vi "Initial Values-format and values-ROI window.vi"() -> (13 "Values.Boolean":bool[](array[boolean]), 14 "Keys setup.DBL":T2=[{"key"="Control FPGA.Clock Freq (MHz)", "Save?"=TRUE, "Default"=240.0}, {"key"="DAQ FPGA.Clock Freq (MHz)", "Save?"=TRUE, "Default"=240.0}], 15 "Values.DBL":dbl[](array[numeric]), 16 "Keys setup.String":T3=[{"key"="Control FPGA.MAC address", "Save?"=TRUE, "Default"="AABBCCDDEEFF"}, {"key"="DAQ FPGA.Target", "Save?"=TRUE, "Default"="RIO0"}, {"key"="XY Stage.COM port", "Save?"=TRUE, "Default"="COM7"}, {"key"="DAQmx Chan.Pockels Control", "Save?"=TRUE, "Default"=""}, {"key"="DAQmx Chan.Hard Shutter", "Save?"=TRUE, "Default"=""}, {"key"="DAQmx Chan.PMT 1", "Save?"=TRUE, "Default"=""}, {"key"="DAQmx Chan.PMT 2", "Save?"=TRUE, "Default"=""}, {"key"="DAQmx Chan.Encoder Trigger", "Save?"=TRUE, "Default"=""}, {"key"="DAQmx Chan.Optional Trigger 1", "Save?"=TRUE, "Default"=""}, {"key"="DAQmx Chan.Optional Trigger 2", "Save?"=TRUE, "Default"=""}, {"key"="DAQmx Chan.Optional Trigger 3", "Save?"=TRUE, "Default"=""}], 17 "Values.Strings":string[](array[string]), 18 "Keys setup.Boolean":T1, 19 "error out":errorcluster)   [LabVIEW 2020]
uses:
  Typedefs/Ini file interface (String).ctl
  Typedefs/Ini file interface (DBL).ctl
  Typedefs/Ini file interface (Boolean).ctl
  User Interface/ROI Entry screen/Globals/gl_ROI Entry UI globals.vi
panel:
  # "NOTES:\n1. \"Control FPGA.Ethernet port\" is detected automatically. It is not saved/loaded from file.\n2. \"Control FPGA.Ethernet Opened\" is detected automatically. It is not saved/loaded from file."
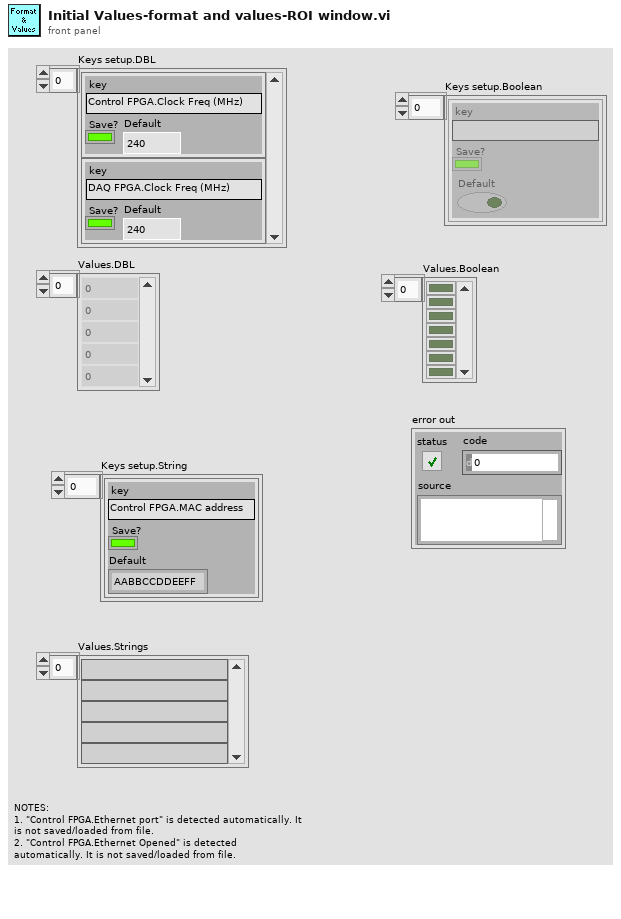
[diagram p1: front panel]
types:
  T1 = typedef "Ini file interface (Boolean).ctl" = cluster{"key":string, "Save?":bool, "Default":bool}[]
  T2 = typedef "Ini file interface (DBL).ctl" = cluster{"key":string, "Save?":bool, "Default":dbl}[]
  T3 = typedef "Ini file interface (String).ctl" = cluster{"key":string, "Save?":bool, "Default":string}[]
  T4 = typedef "ROI entry screen ctrl refs cluster.ctl" = cluster{"Done button":refnum<vi>, "Imaging button":refnum<vi>, "Acquisition button":refnum<vi>, "Scan dwell time per pixel (us)":refnum<vi>, "# of planes":refnum<vi>, "Zoom Ctrl":refnum<vi>, "Equal size":refnum<vi>, "Channel":refnum<vi>, "Image Display":refnum<vi>, "Z-Plane Selector":refnum<vi>, "Number of lines left":refnum<vi>, "Z-stack folder path":refnum<vi>, "POI Density":refnum<vi>, "Arb Plane Entry":refnum<vi>, "Whole Plane":refnum<vi>, "Line Mode":refnum<vi>, "Clear Last":refnum<vi>, "Clear All":refnum<vi>, "Delete Lines":refnum<vi>, "Trial Length (sec)":refnum<vi>, "Palette Type":refnum<vi>, "Intensity slider":refnum<vi>, "# POI":refnum<vi>, "Max Z Proj":refnum<vi>, "Zplane ind":refnum<vi>, "Wavelength (nm)":refnum<vi>, "Number of Trials":refnum<vi>, "Funct stim.trig.enable":refnum<vi>, "Funct stim.trig.delay (s)":refnum<vi>, "Line Mode":refnum<vi>, "Step size (µm)":refnum<vi>, "ROI move mode":refnum<vi>, "Cool-down time (s)":refnum<vi>, "Enable cool-down time":refnum<vi>, "Motor Z ind. (um)":refnum<vi>, "AOL Z ind. (um)":refnum<vi>, "Load Reference Image":refnum<vi>, "Rel.  Res.":refnum<vi>, "ROI LIST":refnum<vi>, "Show All":refnum<vi>, "ROI Type":refnum<vi>, "Start Plane":refnum<vi>, "Stop Plane":refnum<vi>, "Offset ROI":refnum<vi>, "Tab Control":refnum<vi>, "Laser Power(%)":refnum<vi>, "Cycle rate":refnum<vi>, "FOV (Ind.)":refnum<vi>, "Frame Size (Ind.)":refnum<vi>, "Resolution (Ind.)":refnum<vi>, "Pixel Density (Ind)":refnum<vi>, "Laser Power (Ind.)":refnum<vi>, "Dwell Time (Ind.)":refnum<vi>, "Adj MC":refnum<vi>}
  T5 = enum16{"Grayscale", "Binary", "Gradient", "Rainbow", "Temperature", "User Defined"}
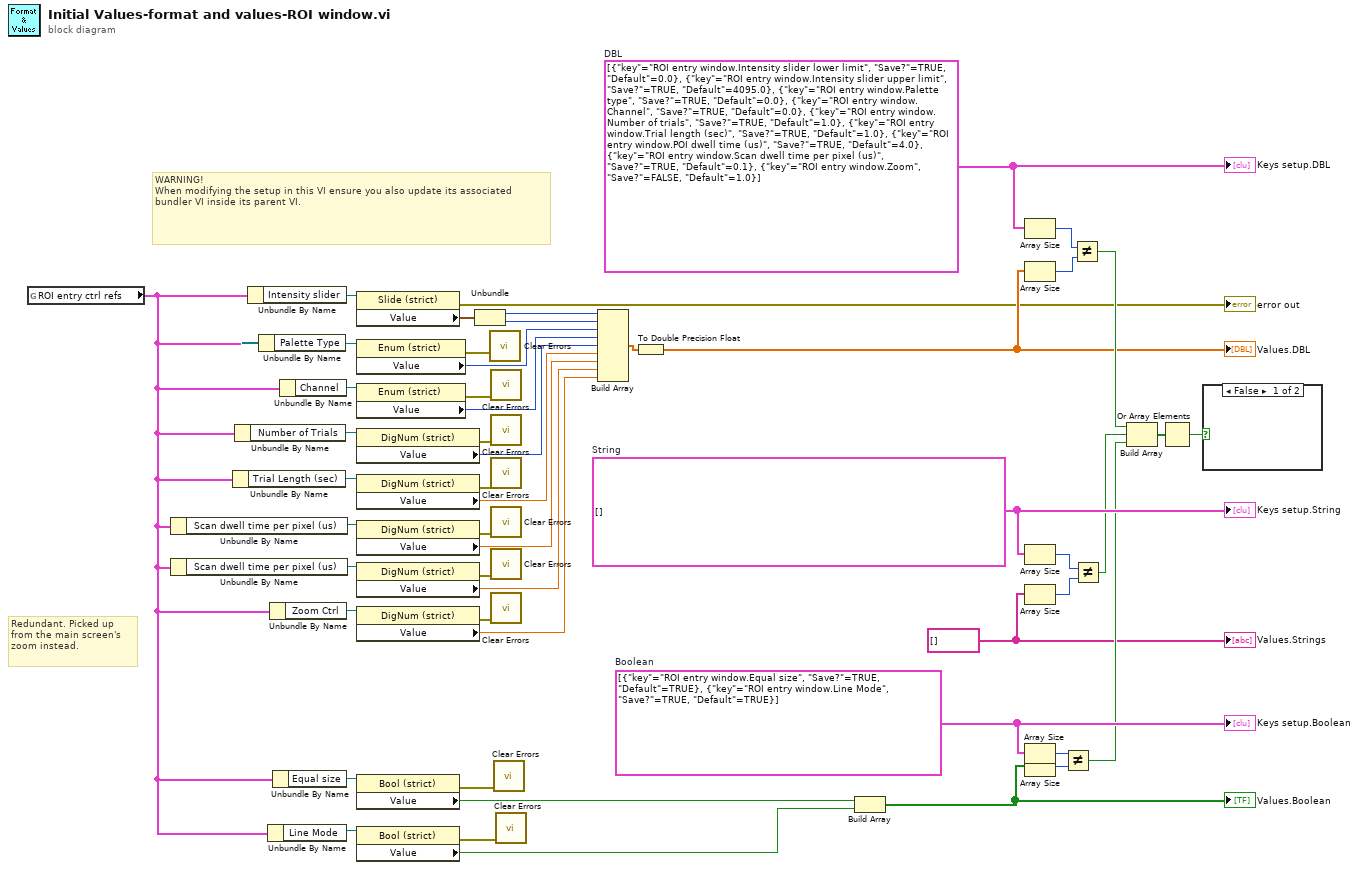
[diagram p0: block diagram]
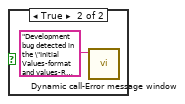
[diagram p2: hidden frame]
diagram:
  w35 = string[] [] ("appended array")
  w48 = T1 [{"key"="ROI entry window.Equal size", "Save?"=TRUE, "Default"=TRUE}, {"key"="ROI entry window.Line Mode", "Save?"=TRUE, "Default"=TRUE}]  # Boolean
  w51 = T3 []  # String
  w50 = T2 [{"key"="ROI entry window.Intensity slider lower limit", "Save?"=TRUE, "Default"=0.0}, {"key"="ROI entry window.Intensity slider upper limit", "Save?"=TRUE, "Default"=4095.0}, {"key"="ROI entry window.Palette type", "Save?"=TRUE, "Default"=0.0}, {"key"="ROI entry window.Channel", "Save?"=TRUE, "Default"=0.0}, {"key"="ROI entry window.Number of trials", "Save?"=TRUE, "Default"=1.0}, {"key"="ROI entry window.Trial length (sec)", "Save?"=TRUE, "Default"=1.0}, {"key"="ROI entry window.POI dwell time (us)", "Save?"=TRUE, "Default"=4.0}, {"key"="ROI entry window.Scan dwell time per pixel (us)", "Save?"=TRUE, "Default"=0.1}, {"key"="ROI entry window.Zoom", "Save?"=FALSE, "Default"=1.0}]  # DBL
  # "Redundant. Picked up from the main screen's zoom instead."
  # "WARNING!\nWhen modifying the setup in this VI ensure you also update its associated bundler VI inside its parent VI."
  n1 = global read "gl_ROI Entry UI globals.vi" "ROI entry ctrl refs"() -> (w4:T4)
  n2 = Unbundle By Name(w4) -> ("Scan dwell time per pixel (us)"=w25:refnum<vi>)
  n3 = Unbundle By Name(w4) -> ("Scan dwell time per pixel (us)"=w5:refnum<vi>)
  n4 = Unbundle By Name(w4) -> ("Trial Length (sec)"=w31:refnum<vi>)
  n5 = Unbundle By Name(w4) -> ("Number of Trials"=w30:refnum<vi>)
  n6 = Unbundle By Name(w4) -> ("Intensity slider"=w26:refnum<vi>)
  n7 = Unbundle By Name(w4) -> ("Palette Type"=w36:refnum<vi>)
  n8 = Unbundle By Name(w4) -> ("Line Mode"=w11:refnum<vi>)
  n9 = Unbundle By Name(w4) -> ("Zoom Ctrl"=w17:refnum<vi>)
  n10 = Unbundle By Name(w4) -> ("Equal size"=w10:refnum<vi>)
  n11 = Unbundle By Name(w4) -> ("Channel"=w33:refnum<vi>)
  n12 = property class="Slide (strict)"(reference=w26) -> (error out=→"error out":errorcluster, "Value"=w24:cluster{i16, i16})  [unwired: 1 in, 1 out]
  n13 = property class="Enum (strict)"(reference=w36) -> (error out=w2:errorcluster, "Value"=w34:T5)  [unwired: 1 in, 1 out]
  n14 = property class="Enum (strict)"(reference=w33) -> (error out=w23:errorcluster, "Value"=w32:enum16{"Green", "Red"})  [unwired: 1 in, 1 out]
  n15 = property class="DigNum (strict)"(reference=w30) -> (error out=w22:errorcluster, "Value"=w29:u16)  [unwired: 1 in, 1 out]
  n16 = property class="DigNum (strict)"(reference=w31) -> (error out=w21:errorcluster, "Value"=w28:dbl)  [unwired: 1 in, 1 out]
  n17 = property class="DigNum (strict)"(reference=w25) -> (error out=w20:errorcluster, "Value"=w19:dbl)  [unwired: 1 in, 1 out]
  n18 = property class="DigNum (strict)"(reference=w5) -> (error out=w6:errorcluster, "Value"=w3:dbl)  [unwired: 1 in, 1 out]
  n19 = property class="DigNum (strict)"(reference=w17) -> (error out=w18:errorcluster, "Value"=w13:dbl)  [unwired: 1 in, 1 out]
  n20 = property class="Bool (strict)"(reference=w10) -> (error out=w9:errorcluster, "Value"=w8:bool)  [unwired: 1 in, 1 out]
  n21 = property class="Bool (strict)"(reference=w11) -> (error out=w12:errorcluster, "Value"=w1:bool)  [unwired: 1 in, 1 out]
  n22 = Unbundle(w24) -> (w15:i16, w14:i16)
  n23 = call <vilib>:"Clear Errors.vi"("error in (no error)"=w2) -> ()  [unwired: 5 in, 2 out]
  n24 = call <vilib>:"Clear Errors.vi"("error in (no error)"=w23) -> ()  [unwired: 5 in, 2 out]
  n25 = call <vilib>:"Clear Errors.vi"("error in (no error)"=w22) -> ()  [unwired: 5 in, 2 out]
  n26 = call <vilib>:"Clear Errors.vi"("error in (no error)"=w21) -> ()  [unwired: 5 in, 2 out]
  n27 = call <vilib>:"Clear Errors.vi"("error in (no error)"=w20) -> ()  [unwired: 5 in, 2 out]
  n28 = call <vilib>:"Clear Errors.vi"("error in (no error)"=w6) -> ()  [unwired: 5 in, 2 out]
  n29 = call <vilib>:"Clear Errors.vi"("error in (no error)"=w18) -> ()  [unwired: 5 in, 2 out]
  n30 = call <vilib>:"Clear Errors.vi"("error in (no error)"=w9) -> ()  [unwired: 5 in, 2 out]
  n31 = call <vilib>:"Clear Errors.vi"("error in (no error)"=w12) -> ()  [unwired: 5 in, 2 out]
  n32 = Build Array(w15, w14, w34, w32, w29, w28, w19, w3, w13) -> (w49:dbl[])
  n33 = To Double Precision Float(number=w49) -> (double precision float=w27:dbl[])
  "Values.DBL" <- w27
  n34 = Build Array(w8, w1) -> (w7:bool[])
  "Values.Boolean" <- w7
  n35 = Array Size(array=w50) -> (size(s)=w45:i32)
  n36 = Array Size(array=w27) -> (size(s)=w44:i32)
  n37 = Array Size(array=w51) -> (size(s)=w47:i32)
  n38 = Array Size(array=w35) -> (size(s)=w46:i32)
  n39 = Array Size(array=w48) -> (size(s)=w43:i32)
  n40 = Array Size(array=w7) -> (size(s)=w42:i32)
  n41 = Not Equal?(x=w43, y=w42) -> (x != y?=w40:bool)
  n42 = Not Equal?(x=w45, y=w44) -> (x != y?=w38:bool)
  n43 = Not Equal?(x=w47, y=w46) -> (x != y?=w37:bool)
  n44 = Build Array(w38, w37, w40) -> (w41:bool[])
  n45 = Or Array Elements(Boolean array=w41) -> (logical OR=w39:bool)
  n46 = case shown="False" w39 {
    frame False {
    }
    frame True {
      n47 = call "Dynamic call-Error message window.vi"("Error Message"="Development bug detected in the \"Initial Values-format and values-ROI window.vi\".\nPlease correct the set up in this VI.") -> ()  [unwired: 10 in, 1 out]
    }
  }
  "Keys setup.String" <- w51
  "Keys setup.DBL" <- w50
  "Values.Strings" <- w35
  "Keys setup.Boolean" <- w48
